vi "Connect.vi"(8 "error in (no error)":errorcluster, 11 "KST101 in":refnum<class "KST101.lvclass">) -> (0 "error out":errorcluster, 3 "KST101 out":refnum<class "KST101.lvclass">)   [LabVIEW 2016, in "Stepper Motor Controller.lvlib" / "KST101.lvclass"]
uses:
  KST101.lvclass
  KST101.lvclass/KST101.ctl
  D:/Workspace/ProCyteOne_LaserModuleAlignment/shared/Thorlabs/Kinesis/Dependencies/Thorlabs.MotionControl.KCube.StepperMotorCLI.dll
  Dependencies/Thorlabs.MotionControl.KCube.StepperMotorCLI.dll
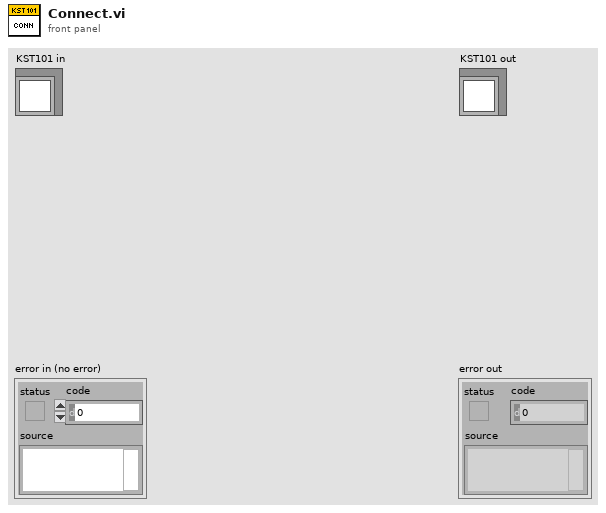
[diagram p1: front panel]
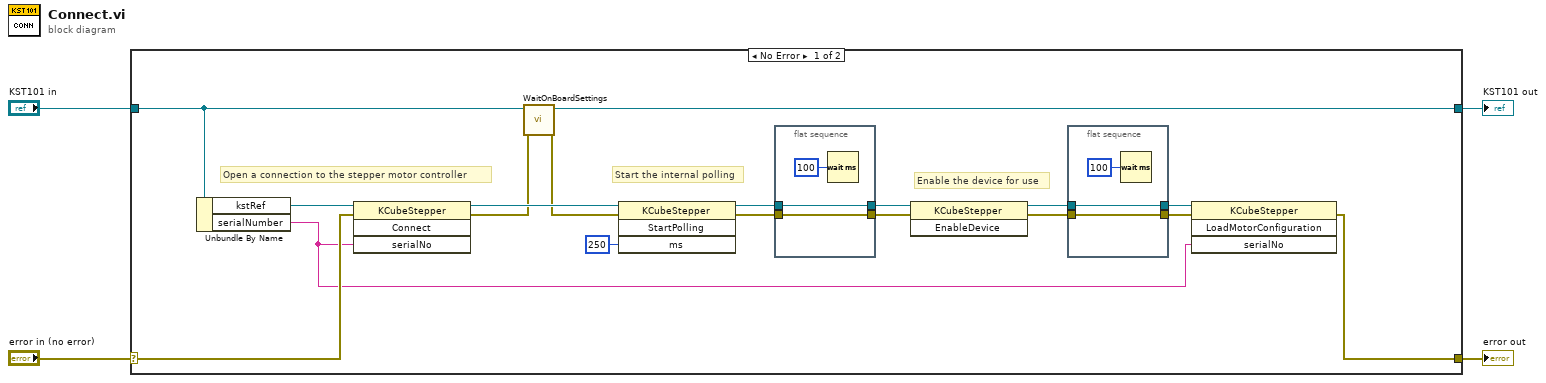
[diagram p0: block diagram]
diagram:
  n1 = case shown="No Error" "error in (no error)" {
    selector: "error in (no error)" -> [w21 w30]
    tunnel: [w6 w30] -> w3
    tunnel: [w17 w29] -> w1
    tunnel: "KST101 in" -> [w18 w29]
    frame No Error {
      # "Enable the device for use"
      # "Start the internal polling"
      # "Open a connection to the stepper motor controller"
      n2 = Unbundle By Name(w18) -> ("kstRef"=w22:refnum<k24>, "serialNumber"=w5:string)
      n3 = invoke class="KCubeStepper" method="Connect"(reference=w22, error in=w21, "serialNo"=w5) -> (reference out=w20:refnum<k24>, error out=w16:errorcluster)  [unwired: 1 in, 2 out]
      n4 = call-dynamic "WaitOnBoardSettings.vi"("error in (no error)"=w16, "KST101 in"=w18) -> ("error out"=w15:errorcluster, "KST101 out"=w17:refnum<class "KST101.lvclass">)  [unwired: 8 in]
      n5 = invoke class="KCubeStepper" method="StartPolling"(reference=w20, error in=w15, "ms"=250) -> (reference out=w11:refnum<k24>, error out=w13:errorcluster)  [unwired: 1 in, 2 out]
      n6 = flat-sequence {
        tunnel: [w28] -> w14
        tunnel: w13 -> [w28]
        tunnel: [w27] -> w12
        tunnel: w11 -> [w27]
        frame #0 {
          n7 = Wait (ms)(milliseconds to wait=u32 100) -> ()  [unwired: 1 out]
        }
      }
      n8 = invoke class="KCubeStepper" method="EnableDevice"(reference=w12, error in=w14) -> (reference out=w9:refnum<k24>, error out=w10:errorcluster)  [unwired: 1 in, 1 out]
      n9 = flat-sequence {
        tunnel: [w25] -> w7
        tunnel: w10 -> [w25]
        tunnel: [w23] -> w8
        tunnel: w9 -> [w23]
        frame #0 {
          n10 = Wait (ms)(milliseconds to wait=u32 100) -> ()  [unwired: 1 out]
        }
      }
      n11 = invoke class="KCubeStepper" method="LoadMotorConfiguration"(reference=w8, error in=w7, "serialNo"=w5) -> (error out=w6:errorcluster)  [unwired: 1 in, 3 out]
    }
    frame Error {
    }
  }
  "error out" <- w3
  "KST101 out" <- w1
